vi "Calc HPF BYTE Size.vi"(9 "Profile Data Point":u16, 10 "Envelope":bool, 11 "Profile Cnt":u8=1) -> (3 "Profile Size":u32)   [LabVIEW 2014, in "Keyence LJ-V7000.lvlib"]
uses:
  Keyence LJ-V7000.lvlib
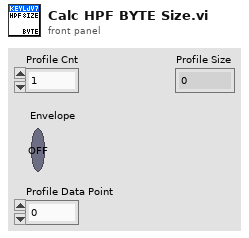
[diagram p1: front panel]
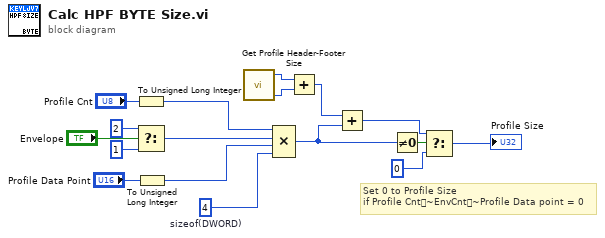
[diagram p0: block diagram]
diagram:
  w9 = u32 4  # sizeof(DWORD)
  # "Set 0 to Profile Size\nif Profile Cnt~EnvCnt~Profile Data point = 0"
  n1 = To Unsigned Long Integer(number="Profile Cnt") -> (unsigned 32bit integer=w12:u32)
  n2 = Select(t=u32 2, s="Envelope", f=u32 1) -> (s? t:f=w11:u32)
  n3 = To Unsigned Long Integer(number="Profile Data Point") -> (unsigned 32bit integer=w10:u32)
  n4 = call "Get Profile Header-Footer Size.vi"() -> ("Footer Size"=w7:u32, "Header Size"=w8:u32)  [unwired: 4 in]
  n5 = Compound Arithmetic op=MULTIPLY(w12, w11, w10, w9) -> (w4:u32)
  n6 = Add(x=w8, y=w7) -> (x+y=w6:u32)
  n7 = Add(x=w6, y=w4) -> (x+y=w3:u32)
  n8 = Not Equal To 0?(x=w4) -> (x != 0?=w5:bool)
  n9 = Select(t=w3, s=w5, f=u32 0) -> (s? t:f=→"Profile Size":u32)
